vi "execute.vi"(8 "error in (no error)":errorcluster, 10 "Context in":refnum<class "Context.lvclass">, 11 "ExitCommand in":refnum<class "ExitCommand.lvclass">) -> (0 "error out":errorcluster, 2 "Context out":refnum<class "Context.lvclass">, 3 "ExitCommand out":refnum<class "ExitCommand.lvclass">)   [LabVIEW 2016, in "ExitCommand.lvclass"]
uses:
  ExitCommand.lvclass
  Context/Context.lvclass
  ExitCommand.lvclass/ExitCommand.ctl
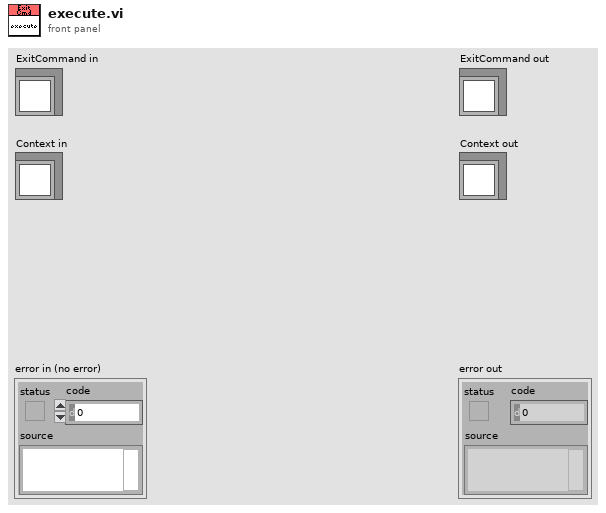
[diagram p1: front panel]
types:
  T1 = typedef "M1M3SupportTopics.lvlib/CommandExit.ctl" = cluster{"CommandId":T2, "Exit":bool}
  T2 = typedef "M1M3SupportTopics.lvlib/CommandId.ctl" = i32
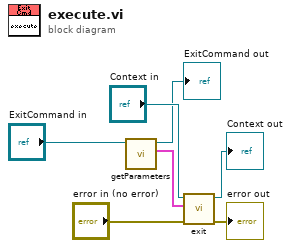
[diagram p0: block diagram]
diagram:
  n1 = call "getParameters.vi"("ExitCommand in"="ExitCommand in") -> ("Parameters"=w7:T1, "ExitCommand out"=→"ExitCommand out":refnum<class "ExitCommand.lvclass">)  [unwired: 9 in]
  n2 = call-dynamic "exit.vi"("error in (no error)"="error in (no error)", "Parameters"=w7, "Context in"="Context in") -> ("error out"=→"error out":errorcluster, "Context out"=→"Context out":refnum<class "Context.lvclass">)  [unwired: 7 in]
